vi "testRunNotCalled.vi"(8 "error in (no error)":errorcluster) -> (0 "error out":errorcluster)   [LabVIEW 2019, in "TestSuiteTest.lvlib" / "Run.lvlib"]
uses:
  Run/Run.lvlib
  TestSuite/TestSuite.lvclass
  TestSuiteTestSupport/TestResultMock/TestResultMock.lvclass
  Assertion/Assertion.lvlib
  C:/Users/de200256/Code/LVUnit/TestResult/TestResult.lvclass
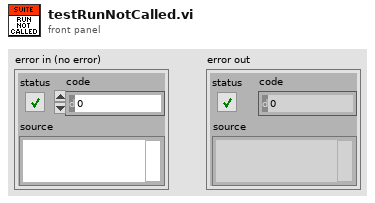
[diagram p1: front panel]
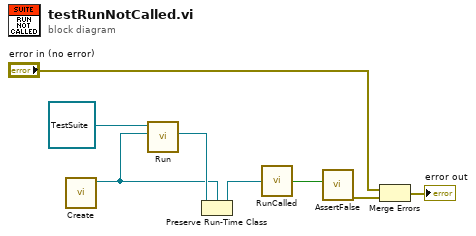
[diagram p0: block diagram]
diagram:
  n1 = call "Create.vi"() -> ("TestResultMock"=w6:refnum<class "TestResultMock.lvclass">)  [unwired: 10 in, 1 out]
  n2 = call-dynamic "Run.vi"("TestResult"=w6, "TestSuite in"=refnum<class "TestSuite.lvclass"> refnum ("TestSuite.lvclass")) -> ("TestResult out"=w7:refnum<class "TestResult.lvclass">)  [unwired: 7 in, 2 out]
  n3 = Preserve Run-Time Class(object in=w7, 2:w6) -> (object out=w5:refnum<class "TestResultMock.lvclass">)  [unwired: 1 in, 1 out]
  n4 = call "RunCalled.vi"("TestResultMock In"=w5) -> ("Run Called"=w4:bool)
  n5 = call "AssertFalse.vi"("Condition"=w4) -> ("error out"=w1:errorcluster)  [unwired: 9 in, 1 out]
  n6 = Merge Errors("error in (no error)", w1) -> (→"error out":errorcluster)
